vi "Raycaster_UpdatePosition.vi"(11 "Game State In":T1) -> (3 "Game State Out":T1)   [LabVIEW 2020]
uses:
  Controls/Game_State.ctl
  Controls/Player_LocationInfo.ctl
  Controls/Player_LocationInfoAxis.ctl
  Controls/Map_Position.ctl
  <vilib>/rvi/FXPMathLib/FxpSinAndCos/subVIs/nifxpmath_SinAndCos_SimConfig.ctl
  <vilib>/rvi/FXPMathLib/FxpSinAndCos/simVIs/DllFxpSinAndCosTemp_sub.vi
  <vilib>/rvi/FXPMathLib/FxpSinAndCos/XNode/nifxpmath_SinAndCos.xnode
  <vilib>/eio/EIONode/EIONode.xnode
  <vilib>/rvi/eio/common/nirviEmuTemplateMethod_errors.vi
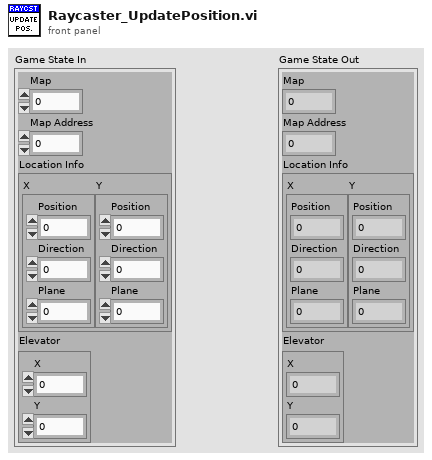
[diagram p1: front panel]
types:
  T1 = typedef "Game_State.ctl" = cluster{"Map":u8, "Map Address":u32, "Location Info":T2, "Elevator":T4}
  T2 = typedef "Player_LocationInfo.ctl" = cluster{"X":T3, "Y":T3}
  T3 = typedef "Player_LocationInfoAxis.ctl" = cluster{"Position":fxp<+/-,32,16>, "Direction":fxp<+/-,32,16>, "Plane":fxp<+/-,32,16>}
  T4 = typedef "Map_Position.ctl" = cluster{"X":fxp<+/-,32,16>, "Y":fxp<+/-,32,16>}
  T5 = enum16{"0", "1", "2", "3", "4", "5", "6", "7", "8", "9", "A", "B", "C", "D", "E", "F", "G", "H", "I", "J", "K", "L", "M", "N", "O", "P", "Q", "R", "S", "T", "U", "V", "W", "X", "Y", "Z", "F1", "F2", "F3", "F4", "F5", "F6", "F7", "F8", "F9", "F10", "F11", "F12", "F13", "F14", "F15", "ADD", "BACK", "BACKSLASH", "CAPITAL", "COMMA", "DECIMAL", "DELETE", "DIVIDE", "DOWN", "END", "EQUALS", "ESCAPE", "GRAVE (`)", "HOME", "INSERT", "LBRACKET", "LCONTROL", "LEFT", "L ALT", "LSHIFT", "LWIN", "MINUS", "MULTIPLY", "NEXT", "NUMLOCK", "NUMPAD_0", "NUMPAD_1", "NUMPAD_2", "NUMPAD_3", "NUMPAD_4", "NUMPAD_5", "NUMPAD_6", "NUMPAD_7", "NUMPAD_8", "NUMPAD_9", "PAUSE", "PERIOD", "PRIOR (PG UP)", "RBRACKET", "RCONTROL", "RETURN", "RIGHT", "R ALT", "RSHIFT", "RWIN", "SCROLL", "SEMICOLON", "SLASH", "SPACE", "SUBTRACT", "TAB", "UP", "ENTER (num pad)", "' (quote)"}[]
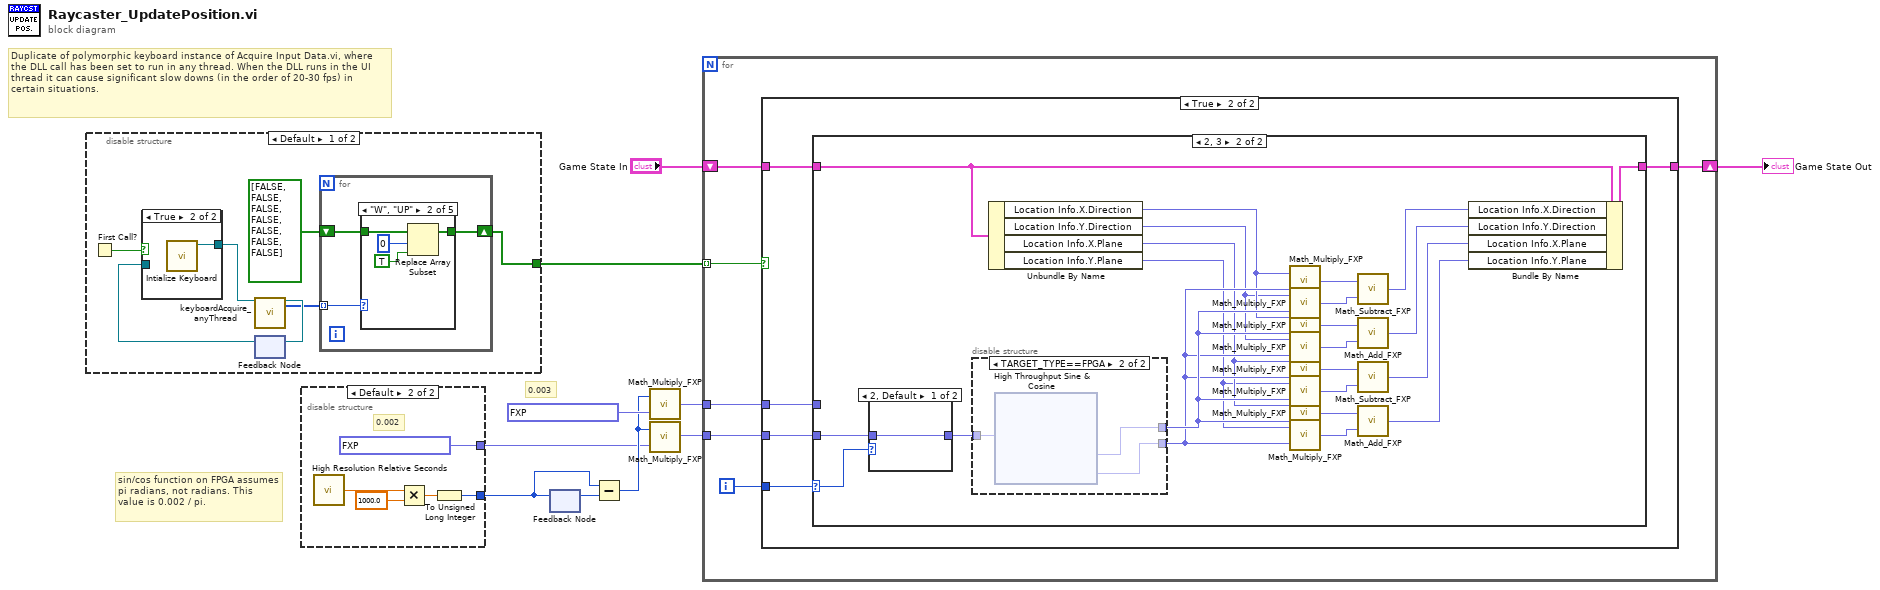
[diagram p0: block diagram]
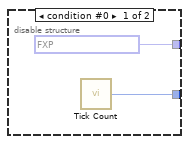
[diagram p2: hidden frame]
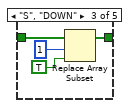
[diagram p4: hidden frame]
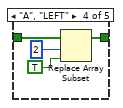
[diagram p5: hidden frame]
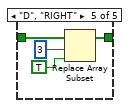
[diagram p6: hidden frame]
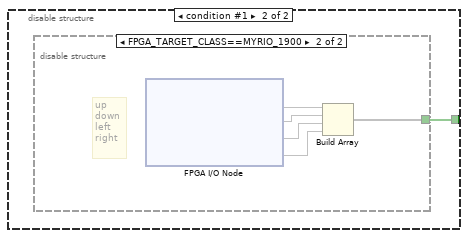
[diagram p8: hidden frame]
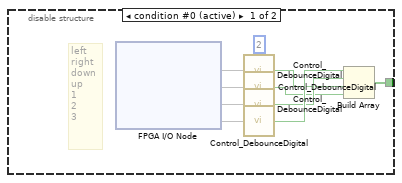
[diagram p9: hidden frame]
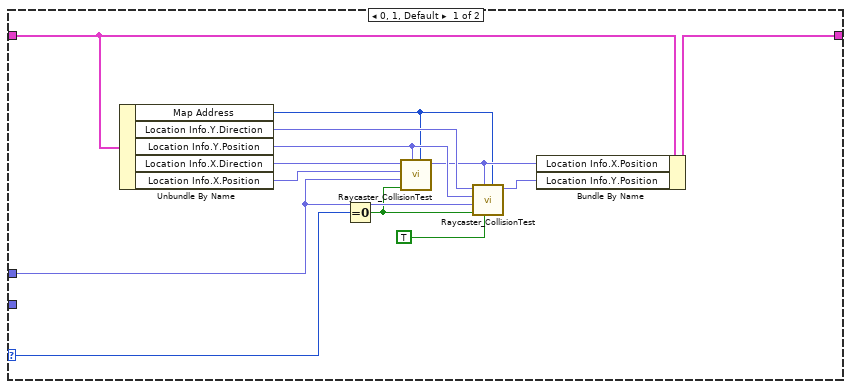
[diagram p11: hidden frame]
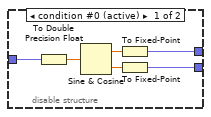
[diagram p12: hidden frame]
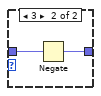
[diagram p13: hidden frame]
diagram:
  # "Duplicate of polymorphic keyboard instance of Acquire Input Data.vi, where the DLL call has been set to run in any thread. When the DLL runs in the UI thread it can cause significant slow downs (in the order of 20-30 fps) in certain situations."
  # "0.003"
  # "sin/cos function on FPGA assumes pi radians, not radians. This value is 0.002 / pi."
  n1 = disable-structure shown="Default" {
    disable-tunnel: [w14 w40] -> w2
    frame condition #0 (active) {
      n2 = First Call?() -> (First Call?: T/F=w17:bool)
      n3 = feedback #1() -> (w16:refnum<k1>)  [unwired: 1 in]
      n4 = case shown="True" w17 {
        tunnel: [w38 w39] -> w13
        tunnel: w16 -> [w38 _]
        frame False {
        }
        frame True {
          n5 = call <vilib>:"Intialize Keyboard.vi"() -> ("device ID"=w39:refnum<k1>)  [unwired: 10 in, 1 out]
        }
      }
      n6 = call "keyboardAcquire_anyThread.vi"("device ID"=w13) -> ("device ID"=w12:refnum<k1>, "keys pressed"=w11:T5)  [unwired: 16 in, 1 out]
      n7 = feedback-in #1(w12) -> ()
      n8 = for {
        shift-right: [w18] -> w14
        shift-left: bool[] [FALSE, FALSE, FALSE, FALSE, FALSE, FALSE, FALSE] -> [w19]
        tunnel: w11 -> [w20] mode=indexing
        n9 = case shown="\"W\", \"UP\"" w20 {
          tunnel: w19 -> [w21 w25 w29 w33 w37]
          tunnel: [w21 w22 w26 w30 w34] -> w18
          frame Default {
          }
          frame "W", "UP" {
            n10 = Replace Array Subset(array=w25, new element=TRUE ("new element/subarray"), index=0) -> (w22:bool[])
          }
          frame "S", "DOWN" {
            n11 = Replace Array Subset(array=w29, new element=TRUE ("new element/subarray"), index=1) -> (w26:bool[])
          }
          frame "A", "LEFT" {
            n12 = Replace Array Subset(array=w33, new element=TRUE ("new element/subarray"), index=2) -> (w30:bool[])
          }
          frame "D", "RIGHT" {
            n13 = Replace Array Subset(array=w37, new element=TRUE ("new element/subarray"), index=3) -> (w34:bool[])
          }
        }
      }
    }
    frame condition #1 {
      n14 = disable-structure shown="FPGA_TARGET_CLASS==MYRIO_1900" {
        disable-tunnel: [w47 w51] -> w40
        frame condition #0 (active) {
          w45 = u16 2 ("Cycles to Filter")
          # "left\nright\ndown\nup\n1\n2\n3"
          n15 = xnode "FPGA I/O Node"() -> ("Mod2/DIO0"=w48, "Mod2/DIO1"=w46, "Mod2/DIO2"=w49, "Mod2/DIO3"=w50)  [unwired: 4 in, 4 out]
          n16 = call "Control_DebounceDigital.vi"("Input Signal"=w48, "Cycles to Filter"=w45) -> ("Output Filtered Signal"=w42:bool)
          n17 = call "Control_DebounceDigital.vi"("Input Signal"=w46, "Cycles to Filter"=w45) -> ("Output Filtered Signal"=w41:bool)
          n18 = call "Control_DebounceDigital.vi"("Input Signal"=w49, "Cycles to Filter"=w45) -> ("Output Filtered Signal"=w43:bool)
          n19 = call "Control_DebounceDigital.vi"("Input Signal"=w50, "Cycles to Filter"=w45) -> ("Output Filtered Signal"=w44:bool)
          n20 = Build Array(w44, w43, w42, w41) -> (w47:bool[])
        }
        frame condition #1 {
          # "up\ndown\nleft\nright"
          n21 = xnode "FPGA I/O Node"() -> ("ConnectorB/DIO0"=w55, "ConnectorB/DIO1"=w54, "ConnectorB/DIO2"=w53, "ConnectorB/DIO3"=w52)  [unwired: 4 in, 4 out]
          n22 = Build Array(w55, w54, w53, w52) -> (w51:void[])
        }
      }
    }
  }
  n23 = disable-structure shown="Default" {
    disable-tunnel: [w57 w59] -> w3
    disable-tunnel: [fxp<+/-,32,16> 0.000640869140625 ("fixed-point type") fxp<+/-,32,16> 0.0019989013671875 ("fixed-point type")] -> w1
    frame condition #0 {
      n24 = call "Tick Count"() -> ("Tick Count(mSec)"=w57:u32)
    }
    frame condition #1 (active) {
      # "0.002"
      n25 = call <vilib>:"High Resolution Relative Seconds.vi"() -> ("relative seconds"=w62:dbl)
      n26 = Multiply(x=w62, y=1000.0) -> (x*y=w60:dbl)
      n27 = To Unsigned Long Integer(number=w60) -> (unsigned 32bit integer=w59:u32)
    }
  }
  n28 = feedback #2() -> (w9:u32)  [unwired: 1 in]
  n29 = feedback-in #2(w3) -> ()
  n30 = Subtract(x=w3, y=w9) -> (x-y=w4:u32)
  n31 = call "Math_Multiply_FXP.vi"("y"=fxp<+/-,32,16> 0.0030059814453125 ("fixed-point type"), "x"=w4) -> ("x*y"=w8:fxp<+/-,32,16>)
  n32 = call "Math_Multiply_FXP.vi"("y"=w1, "x"=w4) -> ("x*y"=w7:fxp<+/-,32,16>)
  n33 = for {
    tunnel: w8 -> [w66]
    shift-right: [w67] -> w6
    shift-left: "Game State In" -> [w68]
    tunnel: w2 -> [w64] mode=indexing
    tunnel: w7 -> [w63]
    i -> [w65]
    n34 = case shown="True" w64 {
      tunnel: w68 -> [w69 w74]
      tunnel: [w69 w73] -> w67
      tunnel: w66 -> [_ w72]
      tunnel: w65 -> [_ w71]
      tunnel: w63 -> [_ w70]
      frame False {
      }
      frame True {
        n35 = case shown="2, 3" w71 {
          selector: w71 -> [w76 w90]
          tunnel: w74 -> [w80 w89]
          tunnel: [w79 w88] -> w73
          tunnel: w72 -> [w78 _]
          tunnel: w70 -> [_ w91]
          frame 0, 1, Default {
            n36 = Unbundle By Name(w80) -> ("Map Address"=w75:u32, "Location Info.Y.Direction"=w85:fxp<+/-,32,16>, "Location Info.Y.Position"=w84:fxp<+/-,32,16>, "Location Info.X.Direction"=w87:fxp<+/-,32,16>, "Location Info.X.Position"=w86:fxp<+/-,32,16>)
            n37 = Equal To 0?(x=w76) -> (x = 0?=w77:bool)
            n38 = call "Raycaster_CollisionTest.vi"("Map Address"=w75, "Other Axis Position"=w84, "Forward?"=w77, "Speed"=w78, "Position"=w86, "Direction"=w87) -> ("New Position"=w83:fxp<+/-,32,16>)  [unwired: 5 in]
            n39 = call "Raycaster_CollisionTest.vi"("Map Address"=w75, "Y Axis (F)"=TRUE ("Y Axis"), "Other Axis Position"=w83, "Forward?"=w77, "Speed"=w78, "Position"=w84, "Direction"=w85) -> ("New Position"=w82:fxp<+/-,32,16>)  [unwired: 4 in]
            n40 = Bundle By Name(cluster=w80, "Location Info.X.Position"=w83, "Location Info.Y.Position"=w82) -> (w79:T1)
          }
          frame 2, 3 {
            n41 = case shown="2, Default" w90 {
              tunnel: w91 -> [w150 w152]
              tunnel: [w150 w151] -> w110
              frame 2, Default {
              }
              frame 3 {
                n42 = Negate(x=w152) -> (-x=w151:fxp<+/-,32,16>)
              }
            }
            n43 = disable-structure shown="TARGET_TYPE==FPGA" {
              disable-tunnel: w110 -> [w116 w119]
              disable-tunnel: [w115 w118] -> w101
              disable-tunnel: [w114 w117] -> w100
              frame condition #0 (active) {
                n44 = To Double Precision Float(number=w116) -> (double precision float=w111:dbl)
                n45 = Sine & Cosine(0:w111) -> (1:w113:dbl, 2:w112:dbl)
                n46 = To Fixed-Point(number=w113) -> (fixed-point=w115:fxp<+/-,32,16>)  [unwired: 1 in]
                n47 = To Fixed-Point(number=w112) -> (fixed-point=w114:fxp<+/-,32,16>)  [unwired: 1 in]
              }
              frame condition #1 {
                n48 = xnode "High Throughput Sine & Cosine"("x (pi)"=w119) -> ("sin(x)"=w118:fxp<+/-,16,2>, "cos(x)"=w117:fxp<+/-,16,2>)
              }
            }
            n49 = Unbundle By Name(w89) -> ("Location Info.X.Direction"=w99:fxp<+/-,32,16>, "Location Info.Y.Direction"=w98:fxp<+/-,32,16>, "Location Info.X.Plane"=w97:fxp<+/-,32,16>, "Location Info.Y.Plane"=w96:fxp<+/-,32,16>)
            n50 = call "Math_Multiply_FXP.vi"("y"=w100, "x"=w99) -> ("x*y"=w109:fxp<+/-,32,16>)
            n51 = call "Math_Multiply_FXP.vi"("y"=w101, "x"=w98) -> ("x*y"=w108:fxp<+/-,32,16>)
            n52 = call "Math_Multiply_FXP.vi"("y"=w101, "x"=w99) -> ("x*y"=w106:fxp<+/-,32,16>)
            n53 = call "Math_Multiply_FXP.vi"("y"=w100, "x"=w98) -> ("x*y"=w107:fxp<+/-,32,16>)
            n54 = call "Math_Multiply_FXP.vi"("y"=w100, "x"=w97) -> ("x*y"=w102:fxp<+/-,32,16>)
            n55 = call "Math_Multiply_FXP.vi"("y"=w101, "x"=w96) -> ("x*y"=w103:fxp<+/-,32,16>)
            n56 = call "Math_Multiply_FXP.vi"("y"=w101, "x"=w97) -> ("x*y"=w105:fxp<+/-,32,16>)
            n57 = call "Math_Multiply_FXP.vi"("y"=w100, "x"=w96) -> ("x*y"=w104:fxp<+/-,32,16>)
            n58 = call "Math_Subtract_FXP.vi"("y"=w108, "x"=w109) -> ("x*y"=w95:fxp<+/-,32,16>)
            n59 = call "Math_Add_FXP.vi"("y"=w107, "x"=w106) -> ("x*y"=w94:fxp<+/-,32,16>)
            n60 = call "Math_Subtract_FXP.vi"("y"=w103, "x"=w102) -> ("x*y"=w93:fxp<+/-,32,16>)
            n61 = call "Math_Add_FXP.vi"("y"=w104, "x"=w105) -> ("x*y"=w92:fxp<+/-,32,16>)
            n62 = Bundle By Name(cluster=w89, "Location Info.X.Direction"=w95, "Location Info.Y.Direction"=w94, "Location Info.X.Plane"=w93, "Location Info.Y.Plane"=w92) -> (w88:T1)
          }
        }
      }
    }
  }
  "Game State Out" <- w6
